vi "zad2.vi"() -> ()   [LabVIEW 2018]
uses:
  <vilib>/Utility/miscctls.llb/LV3DPointTypeDef.ctl
  <vilib>/picture/3D Picture Control/Object/Create Object (drawable).vi
  <vilib>/picture/3D Picture Control/Object/Add Object (reference).vi
  <vilib>/picture/3D Picture Control/NI_3D Picture Control.lvlib
panel:
  out "3D Picture 2":refnum<vi>(3d-picture)
  in  "Scale":T1
  in  "Angle 3":sgl
  in  "Axis 3":T1
  in  "Translation":T1
  out "3D Picture":refnum<vi>(3d-picture)
  in  "stop":bool
  in  "Angle 2":sgl
  in  "Axis 2":T1
  in  "Angle":sgl
  in  "Axis":T1
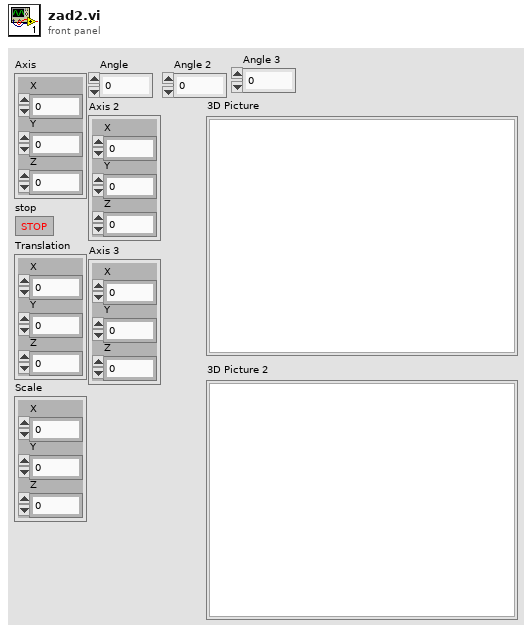
[diagram p1: front panel]
types:
  T1 = typedef "LV3DPointTypeDef.ctl" = cluster{"X":sgl, "Y":sgl, "Z":sgl}
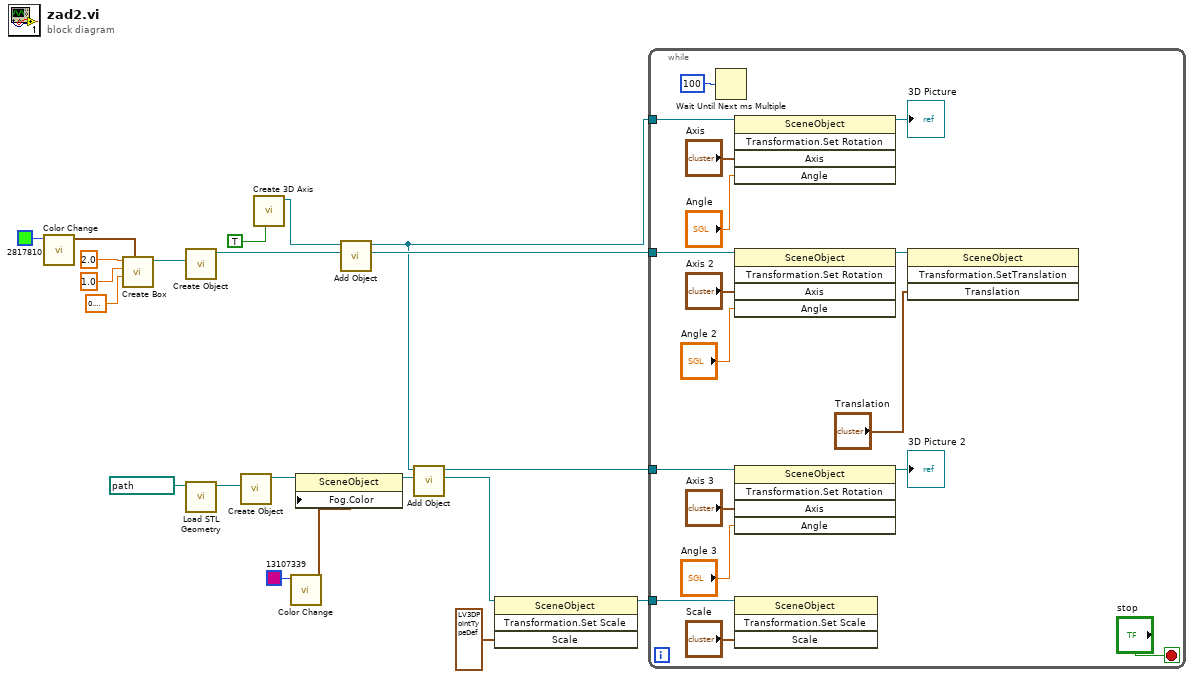
[diagram p0: block diagram]
diagram:
  n1 = call <vilib>:"Color Change.vi"("Color"=u32 2817810) -> ("RGBA"=w5:cluster{"R":sgl, "G":sgl, "B":sgl, "A":sgl})  [unwired: 10 in]
  n2 = call <vilib>:"Create Box.vi"("Color"=w5, "Length Z"=sgl 0.1, "Length Y"=sgl 1.0, "Length X"=sgl 2.0) -> ("New Box Refnum"=w15:refnum<vi>)  [unwired: 6 in, 1 out]
  n3 = call-poly <vilib>:"Create Object.vi"("Geometry"=w15) -> ("Scene:New Object"=w20:refnum<vi>)  [unwired: 9 in, 1 out]
  n4 = call <vilib>:"Load STL Geometry.vi"("Model File"=path "Część3.stl") -> ("New Mesh Refnum"=w12:refnum<vi>)  [unwired: 9 in, 1 out]
  n5 = call-poly <vilib>:"Create Object.vi"("Geometry"=w12) -> ("Scene:New Object"=w4:refnum<vi>)  [unwired: 9 in, 1 out]
  n6 = call <vilib>:"Create 3D Axis.vi"("Axis label?"=TRUE) -> ("New Object Refnum"=w21:refnum<vi>)  [unwired: 9 in, 1 out]
  n7 = call <vilib>:"Color Change.vi"("Color"=u32 13107339) -> ("RGBA"=w2:cluster{"R":sgl, "G":sgl, "B":sgl, "A":sgl})  [unwired: 10 in]
  n8 = property class="SceneObject"(reference=w4, "Fog.Color"=w2) -> (reference out=w3:refnum<vi>)  [unwired: 1 in, 1 out]
  n9 = call-poly <vilib>:"Add Object.vi"("New Object In"=w20, "Scene Object In"=w21) -> ("New Object Out"=w14:refnum<vi>, "Scene Object Out"=w11:refnum<vi>)  [unwired: 7 in, 1 out]
  n10 = call-poly <vilib>:"Add Object.vi"("New Object In"=w3, "Scene Object In"=w11) -> ("New Object Out"=w8:refnum<vi>, "Scene Object Out"=w10:refnum<vi>)  [unwired: 7 in, 1 out]
  n11 = invoke class="SceneObject" method="Transformation.Set Scale"(reference=w8, "Scale"=T1 {"X"=0.2, "Y"=0.2, "Z"=0.2}) -> (reference out=w7:refnum<vi>)  [unwired: 2 in, 3 out]
  n12 = while {
    tunnel: w11 -> [w37]
    tunnel: w14 -> [w38]
    tunnel: w10 -> [w27]
    tunnel: w7 -> [w26]
    stop <- "stop" stop-if-true
    n13 = Wait Until Next ms Multiple(millisecond multiple=u32 100) -> ()  [unwired: 1 out]
    n14 = invoke class="SceneObject" method="Transformation.Set Rotation"(reference=w37, "Axis"="Axis", "Angle"="Angle") -> (reference out=→"3D Picture":refnum<vi>)  [unwired: 2 in, 4 out]
    n15 = invoke class="SceneObject" method="Transformation.Set Rotation"(reference=w38, "Axis"="Axis 2", "Angle"="Angle 2") -> (reference out=w30:refnum<vi>)  [unwired: 2 in, 4 out]
    n16 = invoke class="SceneObject" method="Transformation.Set Rotation"(reference=w27, "Axis"="Axis 3", "Angle"="Angle 3") -> (reference out=→"3D Picture 2":refnum<vi>)  [unwired: 2 in, 4 out]
    n17 = invoke class="SceneObject" method="Transformation.Set Scale"(reference=w26, "Scale"="Scale") -> ()  [unwired: 2 in, 4 out]
    n18 = invoke class="SceneObject" method="Transformation.SetTranslation"(reference=w30, "Translation"="Translation") -> ()  [unwired: 2 in, 4 out]
  }
